vi "Configure Modulation(4FSK).vi"(0 "VISA resource name":refnum<visa-resource-name>, 1 "Enable 4FSK Modulation (F: Disable)":bool, 2 "Hop Frequency 3 (100 Hz)":dbl=100.0, 5 "Channel (1: Channel 1)":i32(ring)=1 items=["Channel 1"=1, "Channel 2"=2], 9 "Hop Frequency 1 (100 Hz)":dbl=100.0, 11 "error in (no error)":errorcluster, 12 "Hop Frequency 2 (100 Hz)":dbl=100.0, 13 "4FSK Rate (100 Hz)":dbl=100.0) -> (4 "VISA resource name out":refnum<visa-resource-name>, 15 "error out":errorcluster)   [LabVIEW 2012, in "RIGOL DG4000 Series.lvlib"]
doc: "Configures 4FSK (4 Frequency Shifting Keying) modulation."
uses:
  <instrlib>/RIGOL DG4000 Series/RIGOL DG4000 Series.lvlib
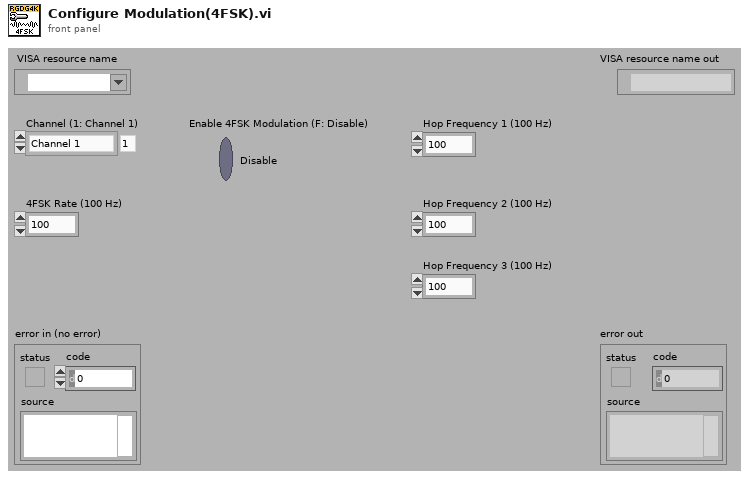
[diagram p1: front panel]
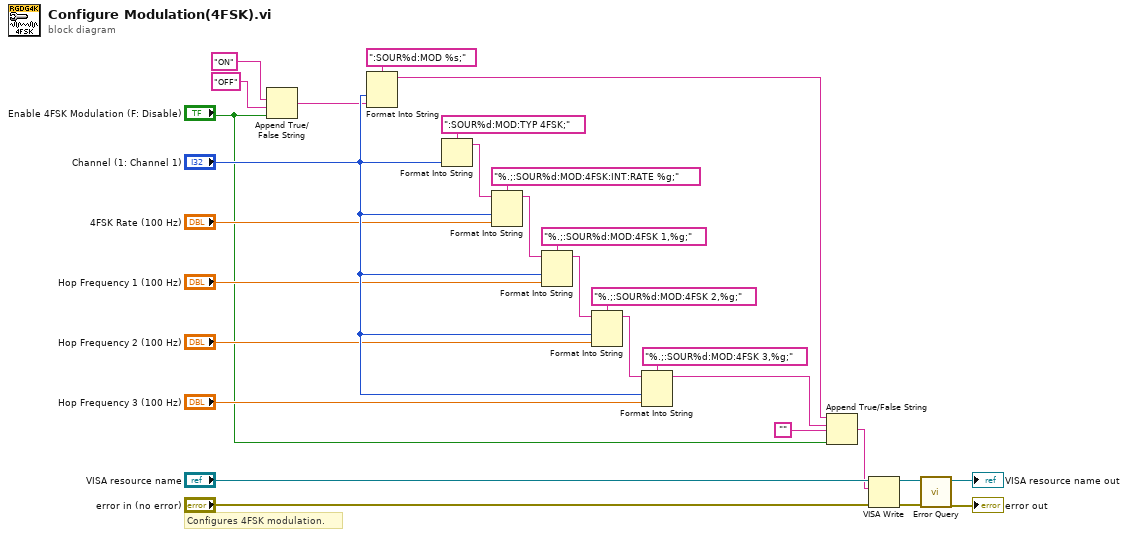
[diagram p0: block diagram]
diagram:
  # "Configures 4FSK modulation."
  n1 = Append True/False String(1:"Enable 4FSK Modulation (F: Disable)", 2:"OFF", 3:"ON") -> (0:w25:string)  [unwired: 1 out]
  n2 = Format Into String(format string=":SOUR%d:MOD %s;", "Channel (1: Channel 1)", w25) -> (resulting string=w5:string)  [unwired: 2 in, 1 out]
  n3 = Format Into String(format string=":SOUR%d:MOD:TYP 4FSK;", "Channel (1: Channel 1)") -> (resulting string=w23:string)  [unwired: 2 in, 1 out]
  n4 = Format Into String(format string="%.;:SOUR%d:MOD:4FSK:INT:RATE %g;", initial string=w23, "Channel (1: Channel 1)", "4FSK Rate (100 Hz)") -> (resulting string=w20:string)  [unwired: 1 in, 1 out]
  n5 = Format Into String(format string="%.;:SOUR%d:MOD:4FSK 1,%g;", initial string=w20, "Channel (1: Channel 1)", "Hop Frequency 1 (100 Hz)") -> (resulting string=w17:string)  [unwired: 1 in, 1 out]
  n6 = Format Into String(format string="%.;:SOUR%d:MOD:4FSK 2,%g;", initial string=w17, "Channel (1: Channel 1)", "Hop Frequency 2 (100 Hz)") -> (resulting string=w14:string)  [unwired: 1 in, 1 out]
  n7 = Format Into String(format string="%.;:SOUR%d:MOD:4FSK 3,%g;", initial string=w14, "Channel (1: Channel 1)", "Hop Frequency 3 (100 Hz)") -> (resulting string=w4:string)  [unwired: 1 in, 1 out]
  n8 = Append True/False String(1:"Enable 4FSK Modulation (F: Disable)", 2:"", 3:w4, 4:w5) -> (0:w1:string)
  n9 = VISA Write(VISA resource name="VISA resource name", write buffer=w1, error in (no error)="error in (no error)") -> (VISA resource name out=w9:refnum<visa-resource-name>, error out=w8:errorcluster)  [unwired: 1 out]
  n10 = call <instrlib>:"Error Query.vi"("error in (no error)"=w8, "VISA resource name"=w9) -> ("error out"=→"error out":errorcluster, "VISA resource name out"=→"VISA resource name out":refnum<visa-resource-name>)  [unwired: 8 out]
